vi "json Parse Float Array - string path.vi"(8 "error in (no error)":errorcluster, 9 "default":sgl[](array[numeric]), 10 "path":string, 11 "JSON Document in":refnum<class "JSON Document.lvclass">) -> (0 "error out":errorcluster, 1 "defaulted?":bool, 2 "value":sgl[](array[numeric]), 3 "JSON Document out":refnum<class "JSON Document.lvclass">, 4 "defaulted indices":i32[](array[numeric]))   [LabVIEW 2015, in "JSON Document.lvclass"]
uses:
  JSON Document.lvclass
  json Parse Float - string path.vi
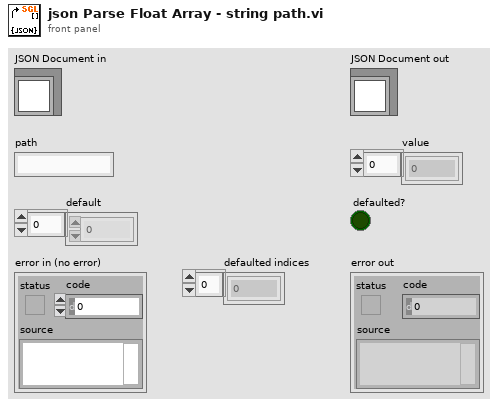
[diagram p1: front panel]
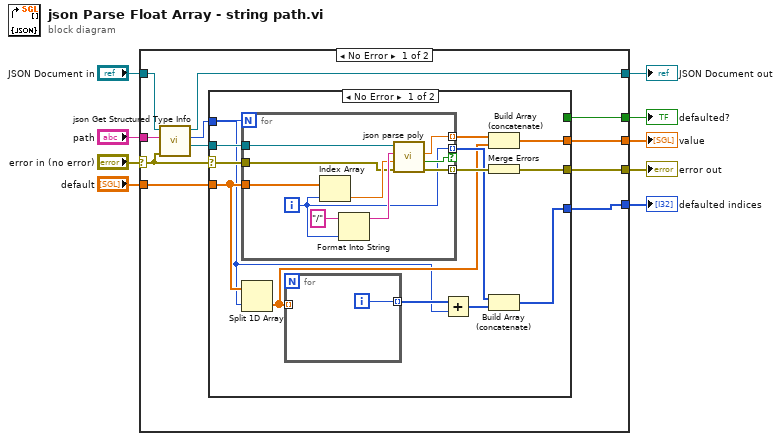
[diagram p0: block diagram]
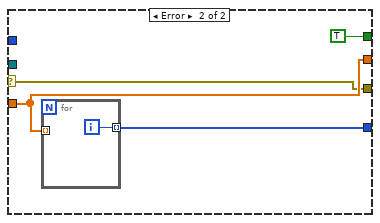
[diagram p2: hidden frame]
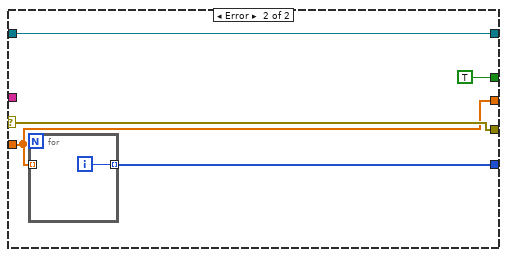
[diagram p3: hidden frame]
diagram:
  n1 = case shown="No Error" "error in (no error)" {
    selector: "error in (no error)" -> [w15 w54]
    tunnel: [w13 w54] -> w4
    tunnel: [w18 w53] -> w2
    tunnel: "JSON Document in" -> [w20 w53]
    tunnel: "default" -> [w14 w52]
    tunnel: "path" -> [w19 _]
    tunnel: [w11 w52] -> w3
    tunnel: [w12 TRUE ("found?")] -> w1
    tunnel: [w10 w51] -> w5
    frame No Error {
      n2 = call "json Get Structured Type Info.vi"("error in (no error)"=w15, "path"=w19, "JSON Document in"=w20) -> ("value out"=w16:refnum<class "JSON Document.lvclass">, "count"=w17:i32, "JSON Document out"=w18:refnum<class "JSON Document.lvclass">)  [unwired: 5 in, 1 out]
      n3 = case shown="No Error" w15 {
        selector: w15 -> [w33 w45]
        tunnel: [w27 w47] -> w11
        tunnel: w17 -> [w22 _]
        tunnel: w14 -> [w29 w47]
        tunnel: [w31 w45] -> w13
        tunnel: w16 -> [w30 _]
        tunnel: [_ TRUE ("found?")] -> w12
        tunnel: [w25 w46] -> w10
        frame No Error {
          n4 = for {
            N: w22 -> [_]
            tunnel: [w38] -> w32 mode=indexing
            tunnel: [w37] -> w28 mode=indexing
            tunnel: w29 -> [w43]
            tunnel: w33 -> [w39]
            tunnel: w30 -> [w42]
            tunnel: [w35] -> w26 mode=indexing if=w36
            i -> [w35]
            n5 = Index Array(array=w43, index=w35) -> (element=w40:sgl)
            n6 = Format Into String(initial string="/", w35) -> (resulting string=w41:string)  [unwired: 2 in, 1 out]
            n7 = call-poly "json parse poly.vi"("error in (no error)"=w39, "default"=w40, "path"=w41, "JSON Document in"=w42) -> ("error out"=w38:errorcluster, "defaulted?"=w36:bool, "value"=w37:sgl)  [unwired: 4 in, 1 out]
          }
          n8 = Split 1D Array(array=w29, index=w22) -> (second subarray=w24:sgl[])  [unwired: 1 out]
          n9 = for {
            tunnel: w24 -> [_] mode=indexing
            tunnel: [w34] -> w23 mode=indexing
            i -> [w34]
          }
          n10 = Add(x=w23, y=w22) -> (x+y=w21:i32[])
          n11 = Build Array (concatenate)(w28, w24) -> (w27:sgl[])
          n12 = Merge Errors(w32) -> (w31:errorcluster)
          n13 = Build Array (concatenate)(w26, w21) -> (w25:i32[])
        }
        frame Error {
          n14 = for {
            tunnel: w47 -> [_] mode=indexing
            tunnel: [w49] -> w46 mode=indexing
            i -> [w49]
          }
        }
      }
    }
    frame Error {
      n15 = for {
        tunnel: [w55] -> w51 mode=indexing
        tunnel: w52 -> [_] mode=indexing
        i -> [w55]
      }
    }
  }
  "error out" <- w4
  "JSON Document out" <- w2
  "value" <- w3
  "defaulted?" <- w1
  "defaulted indices" <- w5
